vi "creat_wave_zero.vi"() -> (0 "添加的数组":waveform(dbl)[](array[waveform]))   [LabVIEW 2018]
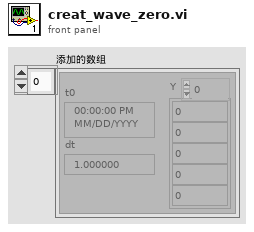
[diagram p1: front panel]
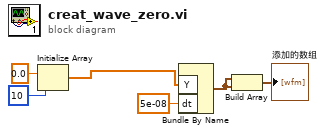
[diagram p0: block diagram]
diagram:
  n1 = Initialize Array(0.0 ("元素"), 10 ("维数大小")) -> (w4:dbl[])
  n2 = Bundle By Name("Y"=w4, "dt"=5e-08) -> (w3:waveform(dbl))  [unwired: 1 in]
  n3 = Build Array(w3, w3) -> (→"添加的数组":waveform(dbl)[])
